vi "PreLoadObjects.vi"(8 "ErrorIn":errorcluster, 11 "ProgressQueue":refnum<queue>) -> (0 "ErrorOut":errorcluster)   [LabVIEW 2021, in "Application.lvclass"]
doc: "Load all objects from the InterfaceConfiguration file into memory"
uses:
  Application.lvclass
  Interface_TAF_IApplicationConfiguration/IApplicationConfiguration/IApplicationConfiguration.lvclass
  5c5df808-c013-4a6b-85e3-bbe17662ba10.vi
  a3facc54-9779-474a-8232-32e1eb8f02f3.vi
  <vilib>/TriekselSoft/TracerLibrary/TracerLibrary/Tracer/protected/SendMessage.vi
  <vilib>/TriekselSoft/TracerLibrary/TracerLibrary/Tracer/protected/Timestamp.vi
  a3facc54-9779-474a-8232-32e1eb8f02f3.vi/f75db090-0877-4668-94fb-75c2140b1617.vi
  <vilib>/TriekselSoft/TracerLibrary/TracerLibrary/Tracer/Tracer_Level-Debug.vi
  <vilib>/TriekselSoft/TracerLibrary/TracerLibrary/Tracer/protected/Tracer_ClassAttributes.vi
  <vilib>/JDP Science/JSONtext/Variant to JSON Text.vi
  <vilib>/JDP Science/JSONtext/LVClass Serializer/JSONtext LVClass Serializer.lvclass
  Application.lvclass/Application.ctl
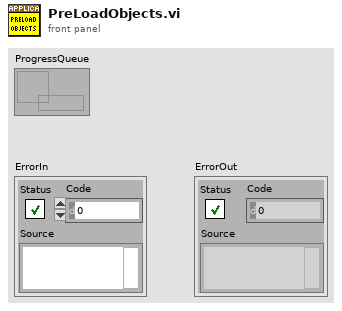
[diagram p1: front panel]
types:
  T1 = cluster{"Not found":cluster{"Name":string, "Path":string}[]}
  T2 = typedef "IApplicationConfiguration.lvclass/ObjectDataDetails.ctl" = cluster{"ObjectName":string, "ObjectType":string, "Interfaces":T3[]}
  T3 = typedef "IApplicationConfiguration.lvclass/ObjectData.ctl" = cluster{"Label":string, "ObjectName":string, "Type":string}
  T4 = typedef "Application.lvclass/ObjectAttributes.ctl" = cluster{"Objects":variant, "BasePath":path, "Application":refnum<class "Application.lvclass">}
  T5 = cluster{"ObjectName":string, "ObjectType":string, "error out":errorcluster}
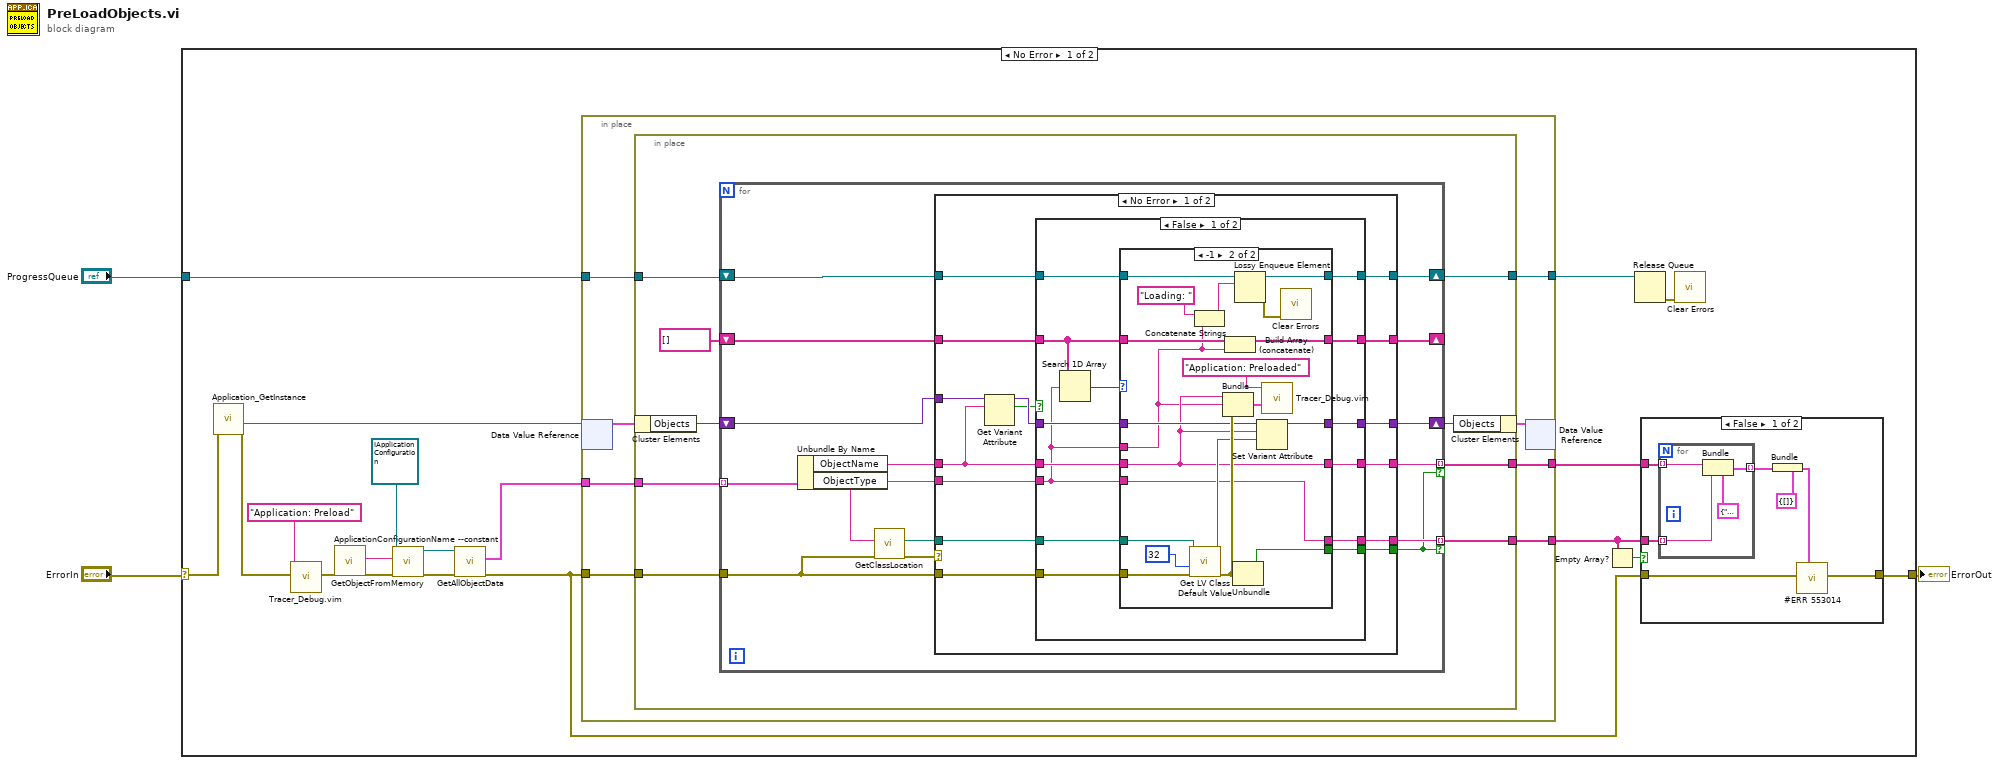
[diagram p0: block diagram]
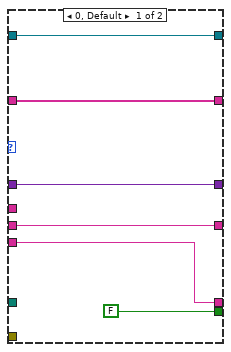
[diagram p2: hidden frame]
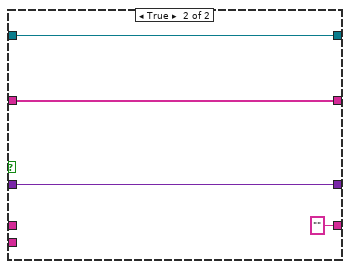
[diagram p3: hidden frame]
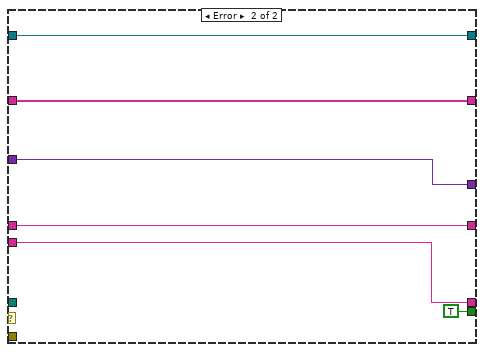
[diagram p4: hidden frame]
diagram:
  n1 = case shown="No Error" "ErrorIn" {
    selector: "ErrorIn" -> [w17 w131]
    tunnel: [w20 w131] -> w2
    tunnel: "ProgressQueue" -> [w6 _]
    frame No Error {
      n2 = call "Application_GetInstance.vi"("ErrorIn"=w17) -> ("ErrorOut"=w16:errorcluster, "DVRRefOut"=w4:refnum<data-value>)  [unwired: 6 in, 3 out]
      n3 = call "Tracer_Debug.vim"("Error In"=w16, "Text"="Application: Preload") -> ("Error Out"=w19:errorcluster)  [unwired: 9 in]
      n4 = call "ApplicationConfigurationName --constant.vi"() -> ("AppConfigName"=w13:string)  [unwired: 10 in, 1 out]
      n5 = call "GetObjectFromMemory.vi"("ErrorIn"=w19, "ObjectName"=w13, "Type"=refnum<class "IApplicationConfiguration.lvclass"> refnum ("IApplicationStructure")) -> ("ErrorOut"=w21:errorcluster, "ObjectOut"=w12:refnum<class "IApplicationConfiguration.lvclass">)  [unwired: 7 in]
      n6 = call-dynamic "GetAllObjectData.vi"("ErrorIn"=w21, "ReferenceIn"=w12) -> ("ErrorOut"=w15:errorcluster, "Objects"=w11:T2[])  [unwired: 7 in, 1 out]
      n7 = in-place {
        in-place-border: w11 -> [w28]
        in-place-border: w15 -> [w29]
        in-place-border: [w27] -> w9
        in-place-border: [w26] -> w8
        in-place-border: w6 -> [w25]
        in-place-border: [w24] -> w5
        n8 = in-place-dvr #1(w4) -> (w23:T4)  [unwired: 1 out]
        n9 = in-place {
          in-place-border: w28 -> [w37]
          in-place-border: w29 -> [w38]
          in-place-border: [w36] -> w27
          in-place-border: [w35] -> w26
          in-place-border: w25 -> [w33]
          in-place-border: [w32] -> w24
          n10 = in-place-cluster #2(w23) -> ("Objects"=w31:variant)
          n11 = for {
            tunnel: w38 -> [w53]
            tunnel: w37 -> [w43] mode=indexing
            tunnel: [w40] -> w36 mode=indexing if=w39
            tunnel: [w51] -> w35 mode=indexing if=w39
            shift-right: [w49] -> _
            shift-left: string[] [] -> [w50]
            shift-right: [w47] -> w32
            shift-left: w33 -> [w48]
            shift-right: [w45] -> w30
            shift-left: w31 -> [w46]
            n12 = Unbundle By Name(w43) -> ("ObjectName"=w44:string, "ObjectType"=w42:string)
            n13 = call "GetClassLocation.vi"("ErrorIn"=w53, "ClassString"=w42) -> ("ErrorOut"=w52:errorcluster, "ClassFilePath"=w41:path)  [unwired: 8 in]
            n14 = case shown="No Error" w52 {
              tunnel: w41 -> [w67 _]
              tunnel: [w66 w115] -> w51
              tunnel: w50 -> [w65 w117]
              tunnel: [w64 w117] -> w49
              tunnel: w48 -> [w63 w118]
              tunnel: [w62 w118] -> w47
              tunnel: w46 -> [w61 w116]
              tunnel: [w60 w116] -> w45
              tunnel: w44 -> [w57 w115]
              tunnel: w53 -> [w68 _]
              tunnel: w42 -> [w56 w114]
              tunnel: [w55 w114] -> w40
              tunnel: [w54 TRUE ("status")] -> w39
              frame No Error {
                n15 = Get Variant Attribute(Variant=w61, name=w57) -> (duplicate Variant=w59:variant, found=w58:bool)  [unwired: 2 in, 2 out]
                n16 = case shown="False" w58 {
                  tunnel: w68 -> [w82 _]
                  tunnel: w67 -> [w81 _]
                  tunnel: [w80 _] -> w54
                  tunnel: w65 -> [w78 w111]
                  tunnel: [w77 w111] -> w64
                  tunnel: w57 -> [w76 _]
                  tunnel: [w75 "" ("TargetObjectName")] -> w66
                  tunnel: w63 -> [w74 w112]
                  tunnel: [w73 w112] -> w62
                  tunnel: w59 -> [w72 w110]
                  tunnel: [w71 w110] -> w60
                  tunnel: w56 -> [w69 _]
                  tunnel: [w70 _] -> w55
                  frame False {
                    n17 = Search 1D Array(1D array=w78, element=w69) -> (index of element=w79:i32)  [unwired: 1 in]
                    n18 = case shown="-1" w79 {
                      tunnel: w82 -> [_ w108]
                      tunnel: w81 -> [_ w105]
                      tunnel: [FALSE ("status") w104] -> w80
                      tunnel: w78 -> [w85 w100]
                      tunnel: w69 -> [_ w90]
                      tunnel: [w85 w99] -> w77
                      tunnel: w76 -> [w87 w91]
                      tunnel: [w87 w91] -> w75
                      tunnel: w74 -> [w86 w98]
                      tunnel: [w86 w97] -> w73
                      tunnel: w72 -> [w84 w96]
                      tunnel: [w84 w94] -> w71
                      tunnel: [w83 w89] -> w70
                      tunnel: w69 -> [w83 w89]
                      frame 0, Default {
                      }
                      frame -1 {
                        n19 = call <vilib>:"Get LV Class Default Value.vi"("error in (no error)"=w108, "options"=u32 32, "class path"=w105) -> ("error out"=w106:errorcluster, "object"=w95:refnum<class>)  [unwired: 7 in]
                        n20 = Concatenate Strings("Loading: " ("string"), w90) -> (w102:string)
                        n21 = Bundle("ObjectName"=w91, "ObjectType"=w90, "error out"=w106) -> (w92:T5)  [unwired: 1 in]
                        n22 = Build Array (concatenate)(w100, w90) -> (w99:string[])
                        n23 = Unbundle(w106) -> ("status"=w104:bool)  [unwired: 2 out]
                        n24 = Lossy Enqueue Element(queue=w98, element=w102) -> (queue out=w97:refnum<queue>, error out=w107:errorcluster)  [unwired: 1 in, 2 out]
                        n25 = Set Variant Attribute(Variant=w96, name=w91, value=w95) -> (Variant out=w94:variant)  [unwired: 1 in, 2 out]
                        n26 = call "Tracer_Debug.vim"("Data"=w92, "Text"="Application: Preloaded") -> ()  [unwired: 9 in, 1 out]
                        n27 = call <vilib>:"Clear Errors.vi"("error in (no error)"=w107) -> ()  [unwired: 5 in, 2 out]
                      }
                    }
                  }
                  frame True {
                  }
                }
              }
              frame Error {
              }
            }
          }
          n28 = in-place-cluster #2("Objects"=w30) -> (w22:T4)
        }
        n29 = in-place-dvr #1(w22) -> ()  [unwired: 2 out]
      }
      n30 = Empty Array?(array=w9) -> (empty?=w10:bool)
      n31 = Release Queue(queue=w5) -> (error out=w18:errorcluster)  [unwired: 2 in, 2 out]
      n32 = case shown="False" w10 {
        tunnel: w9 -> [w123 _]
        tunnel: w15 -> [w125 w130]
        tunnel: [w124 w130] -> w20
        tunnel: w8 -> [w122 _]
        frame False {
          n33 = for {
            tunnel: w123 -> [w127] mode=indexing
            tunnel: w122 -> [w128] mode=indexing
            tunnel: [w126] -> w121 mode=indexing
            n34 = Bundle(cluster=cluster{"Name":string, "Type":string} {"Name"="", "Type"=""}, "Name"=w128, "Type"=w127) -> (w126:cluster{"Name":string, "Type":string})
          }
          n35 = Bundle(cluster=T1 {"Not found"=[]}, "Not found"=w121) -> (w120:T1)
          n36 = call "#ERR 553014"("Data"=w120, "error in (no error)"=w125) -> ("error out"=w124:errorcluster)  [unwired: 9 in]
        }
        frame True {
        }
      }
      n37 = call <vilib>:"Clear Errors.vi"("error in (no error)"=w18) -> ()  [unwired: 5 in, 2 out]
    }
    frame Error {
    }
  }
  "ErrorOut" <- w2
